vi "roc.vi"() -> ()   [LabVIEW 2019]
panel:
  in  "File Path (OCR/OCV 1)":path=path "D:/3下課程/總結式課程/影像/OCR/train1.abc"
  out "Image Out":T1(plugin-control)
  out "Image":T1(plugin-control)
  out "String (OCR/OCV 1)":string
  in  "Stop (F)":bool
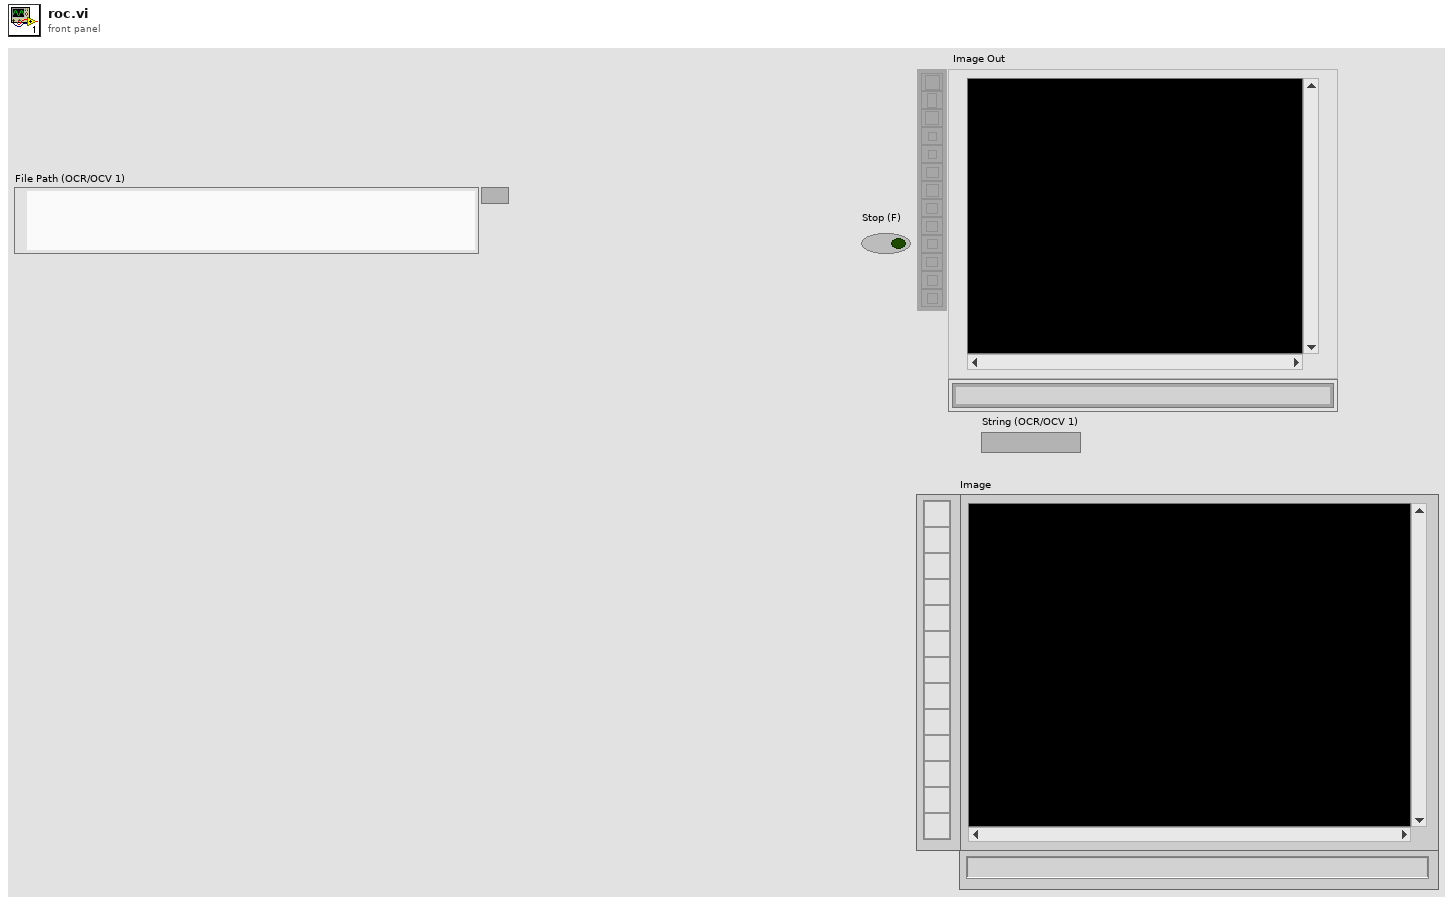
[diagram p1: front panel]
types:
  T1 = typedef "IMAQ Image.ctl" = refnum<image>
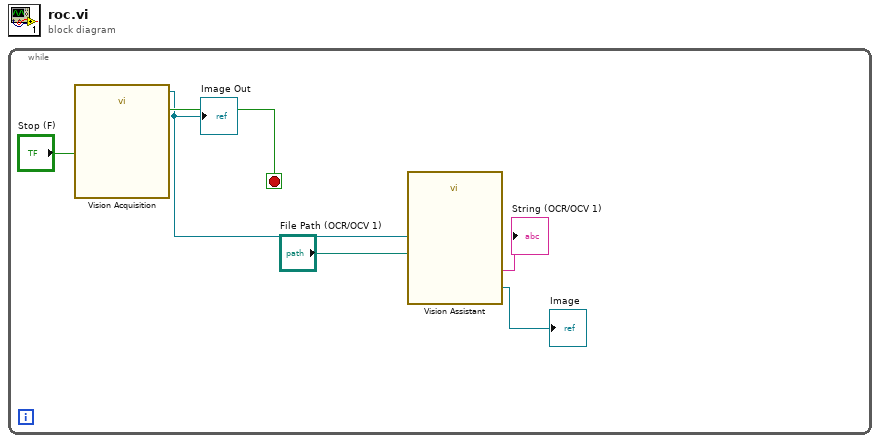
[diagram p0: block diagram]
diagram:
  n1 = while {
    stop <- w5 stop-if-true
    n2 = call "Vision Acquisition"("Stop (F)"="Stop (F)") -> ("Image Out"=w3:T1, "Stopped"=w5:bool)  [unwired: 23 in, 2 out]
    "Image Out" <- w3
    n3 = call "Vision Assistant"("Image In"=w3, "File Path (OCR/OCV 1)"="File Path (OCR/OCV 1)") -> ("Image Out"=→"Image":T1, "String (OCR/OCV 1)"=→"String (OCR/OCV 1)":string)  [unwired: 23 in, 1 out]
  }
